vi "Write Cell.vi"(8 "error in":errorcluster, 9 "Mediçao":dbl, 10 "Cell Name":string, 11 "NI_report in":refnum<class "NI_report.lvclass">) -> (0 "error out":errorcluster, 3 "NI_report out":refnum<class "NI_report.lvclass">)   [LabVIEW 2015]
uses:
  <vilib>/Utility/NIReport.llb/NI_report.lvclass
  <vilib>/Utility/NIReport.llb/Append Report Text (str wrap).vi
  <vilib>/addons/_office/NI_ReportGenerationToolkit.lvlib
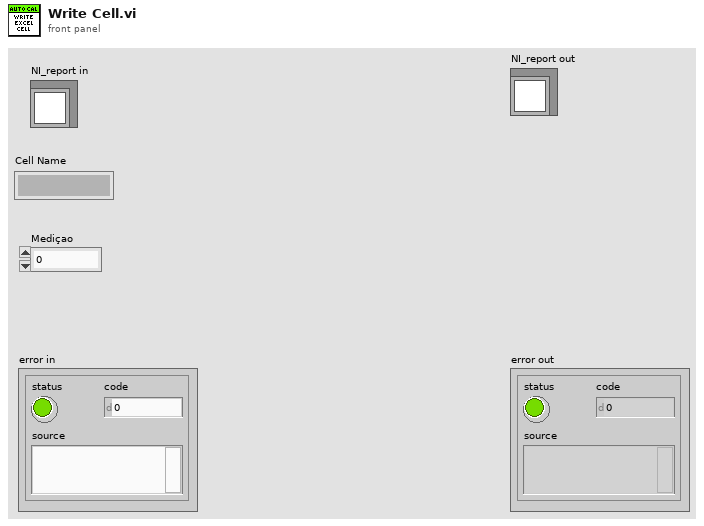
[diagram p1: front panel]
types:
  T1 = cluster{"position (excel)":cluster{"row":i32, "column":i32}, "name (excel)":string, "bookmark (word)":string}
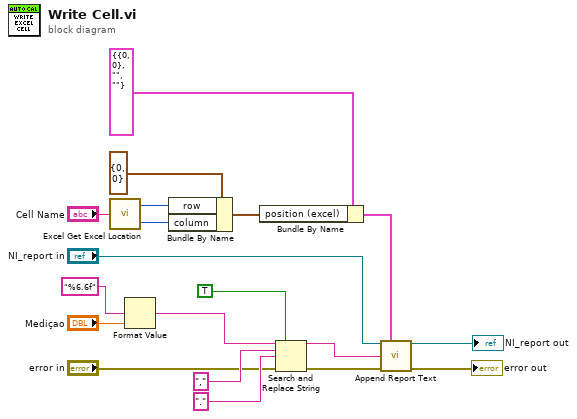
[diagram p0: block diagram]
diagram:
  n1 = call <vilib>:"Excel Get Excel Location.vi"("cell's name"="Cell Name") -> ("row"=w14:i32, "column"=w15:i32)
  n2 = Format Value(format string="%6.6f", value (0)="Mediçao") -> (output string=w7:string)  [unwired: 1 in]
  n3 = Bundle By Name(cluster=cluster{"row":i32, "column":i32} {"row"=0, "column"=0} ("position (excel)"), "row"=w14, "column"=w15) -> (w16:cluster{"row":i32, "column":i32})
  n4 = Bundle By Name(cluster=T1 {"position (excel)"={"row"=0, "column"=0}, "name (excel)"="", "bookmark (word)"=""} ("MS Office parameters"), "position (excel)"=w16) -> (w17:T1)
  n5 = Search and Replace String(replace all?=TRUE ("replace all? (F)"), input string=w7, search string=",", replace string="." ("replace string (\"\")"), error in="error in") -> (result string=w3:string, error out=w2:errorcluster)  [unwired: 3 in, 2 out]
  n6 = call-poly <vilib>:"Append Report Text.vi"("report in"="NI_report in", "MS Office parameters"=w17, "text"=w3, "error in (no error)"=w2) -> ("report out"=→"NI_report out":refnum<class "NI_report.lvclass">, "error out"=→"error out":errorcluster)  [unwired: 8 in, 2 out]
